vi "thcd_get_samp.vi"(6 "err_in":errorcluster, 7 "thcd_visa":refnum<visa-resource-name>, 8 "thcd_com":T1(ring), 9 "thcd_ch":T2, 10 "thcd_b2r":u32, 11 "thcd_delay":u32=500) -> (0 "thcd_st":bool, 1 "thcd_res_msg":string, 2 "thcd_res_str":string, 3 "thcd_res":dbl, 4 "err_out":errorcluster, 5 "thcd_visa":refnum<visa-resource-name>)   [LabVIEW 2018, in "1039_mod.lvlib"]
uses:
  thcd_controls/ctrl_chn_thcd.ctl
  1039_mod/1039_mod.lvlib
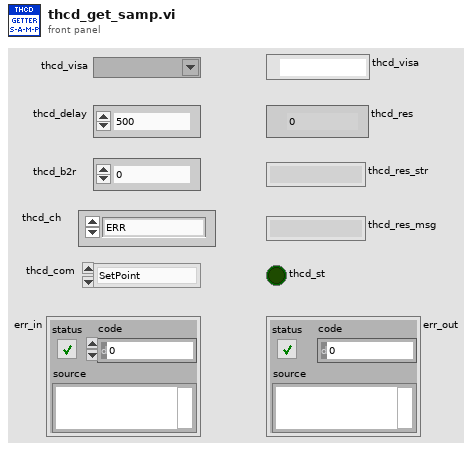
[diagram p1: front panel]
types:
  T1 = enum16{"SetPoint", "AlarmH", "AlarmL", "Multiplier", "CalibValue"}
  T2 = typedef "ctrl_chn_thcd.ctl" = enum8{"ERR", "1", "2", "3", "4"}
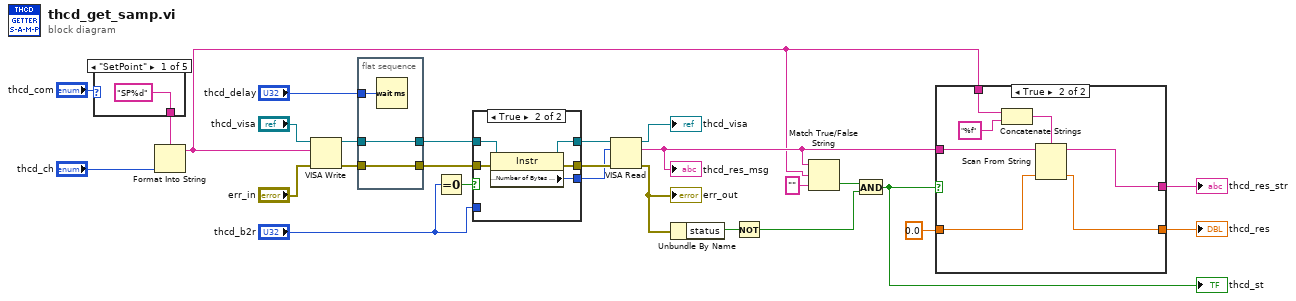
[diagram p0: block diagram]
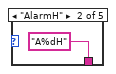
[diagram p2: hidden frame]
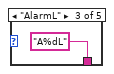
[diagram p3: hidden frame]
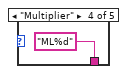
[diagram p4: hidden frame]
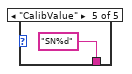
[diagram p5: hidden frame]
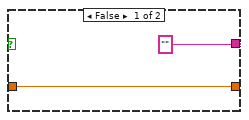
[diagram p7: hidden frame]
diagram:
  n1 = case shown="\"SetPoint\"" "thcd_com" {
    tunnel: ["SP%d" ("format string") "A%dH" ("format string") "A%dL" ("format string") "ML%d" ("format string") "SN%d" ("format string")] -> w1
    frame "SetPoint" {
    }
    frame "AlarmH" {
    }
    frame "AlarmL" {
    }
    frame "Multiplier" {
    }
    frame "CalibValue" {
    }
  }
  n2 = Format Into String(format string=w1, "thcd_ch") -> (resulting string=w9:string)  [unwired: 2 in, 1 out]
  n3 = VISA Write(VISA resource name="thcd_visa", write buffer=w9, error in (no error)="err_in") -> (VISA resource name out=w25:refnum<visa-resource-name>, error out=w27:errorcluster)  [unwired: 1 out]
  n4 = flat-sequence {
    tunnel: w27 -> [w34]
    tunnel: [w34] -> w26
    tunnel: w25 -> [w33]
    tunnel: [w33] -> w24
    tunnel: "thcd_delay" -> [w35]
    frame #0 {
      n5 = Wait (ms)(milliseconds to wait=w35) -> ()  [unwired: 1 out]
    }
  }
  n6 = Equal To 0?(x="thcd_b2r") -> (x = 0?=w6:bool)
  n7 = case shown="True" w6 {
    tunnel: w26 -> [w37 w43]
    tunnel: w24 -> [w38 w42]
    tunnel: [w38 w41] -> w23
    tunnel: [w37 w40] -> w22
    tunnel: [w36 w39] -> w5
    tunnel: "thcd_b2r" -> [w36 _]
    frame False {
    }
    frame True {
      n8 = property class="Instr"(reference=w42, error in=w43) -> (reference out=w41:refnum<visa-resource-name>, error out=w40:errorcluster, "Serial Settings:Number of Bytes at Serial Port"=w39:u32)
    }
  }
  n9 = VISA Read(VISA resource name=w23, byte count=w5, error in (no error)=w22) -> (VISA resource name out=→"thcd_visa":refnum<visa-resource-name>, read buffer=w15:string, error out=w16:errorcluster)  [unwired: 1 out]
  "err_out" <- w16
  "thcd_res_msg" <- w15
  n10 = Unbundle By Name(w16) -> ("status"=w13:bool)
  n11 = Not(x=w13) -> (.not. x?=w11:bool)
  n12 = Match True/False String(2:"" ("false string"), 3:w9, 4:w15) -> (0:w12:bool)  [unwired: 1 out]
  n13 = And(x=w12, y=w11) -> (x .and. y?=w10:bool)
  "thcd_st" <- w10
  n14 = case shown="True" w10 {
    tunnel: w15 -> [_ w50]
    tunnel: w9 -> [_ w49]
    tunnel: [w44 w48] -> w8
    tunnel: ["" w47] -> w7
    tunnel: 0.0 -> [w44 w46]
    frame False {
    }
    frame True {
      n15 = Concatenate Strings(w49, "%f" ("string")) -> (w51:string)
      n16 = Scan From String(format string=w51, input string=w50, default 1=w46) -> (remaining string=w47:string, output 1=w48:dbl)  [unwired: 2 in, 2 out]
    }
  }
  "thcd_res_str" <- w7
  "thcd_res" <- w8
